vi "9205_UI.vi"(8 "error in (no error)":errorcluster, 11 "Node Ptr":T2 format="%.0x") -> (0 "error out":errorcluster)   [LabVIEW 2017, in "Modules.lvlib" / "9205.lvclass"]
uses:
  9205.lvclass
  <vilib>/NI Veristand/Custom Device API/Custom Device Item Ref.ctl
  RSI Module/SubPanel Command.ctl
  C:/Users/dbuck/Documents/GitHub/Scan-Engine-Custom-Device-Classes/Source/RSI Module/RSI Module.lvclass
  9205.lvclass/9205.ctl
  Range.ctl
  Terminal mode.ctl
  RSI Module/RSI Module.lvclass
  <vilib>/NI Veristand/Custom Device API/Custom Device API.lvlib
panel:
  in  "_Update Chan Settings":bool
  in  "_Update Ring Controls":bool
  in  "_Voltage Ranges":T1(array[ring])=[enum."+/- 10V", enum."+/- 10V", enum."+/- 10V", enum."+/- 10V", enum."+/- 10V", enum."+/- 10V", enum."+/- 10V", enum."+/- 10V", enum."+/- 10V", enum."+/- 10V", enum."+/- 10V", enum."+/- 10V", enum."+/- 10V", enum."+/- 10V", enum."+/- 10V", enum."+/- 10V", enum."+/- 10V", enum."+/- 10V", enum."+/- 10V", enum."+/- 10V", enum."+/- 10V", enum."+/- 10V", enum."+/- 10V", enum."+/- 10V", enum."+/- 10V", enum."+/- 10V", enum."+/- 10V", enum."+/- 10V", enum."+/- 10V", enum."+/- 10V", enum."+/- 10V", enum."+/- 10V"]
  in  "_Terminal Modes":enum8{"RSE", "NRSE", "DIFF"}[](array[ring])=[enum."RSE", enum."RSE", enum."RSE", enum."RSE", enum."RSE", enum."RSE", enum."RSE", enum."RSE", enum."RSE", enum."RSE", enum."RSE", enum."RSE", enum."RSE", enum."RSE", enum."RSE", enum."RSE", enum."RSE", enum."RSE", enum."RSE", enum."RSE", enum."RSE", enum."RSE", enum."RSE", enum."RSE", enum."RSE", enum."RSE", enum."RSE", enum."RSE", enum."RSE", enum."RSE", enum."RSE", enum."RSE"]
  out "_SupportedRanges":string[][](array[string])=[["+/- 10V", "+/- 5V", "+/- 1V", "+/- 200mV"], ["+/- 10V", "+/- 5V", "+/- 1V", "+/- 200mV"], ["+/- 10V", "+/- 5V", "+/- 1V", "+/- 200mV"], ["+/- 10V", "+/- 5V", "+/- 1V", "+/- 200mV"], ["+/- 10V", "+/- 5V", "+/- 1V", "+/- 200mV"], ["+/- 10V", "+/- 5V", "+/- 1V", "+/- 200mV"], ["+/- 10V", "+/- 5V", "+/- 1V", "+/- 200mV"], ["+/- 10V", "+/- 5V", "+/- 1V", "+/- 200mV"], ["+/- 10V", "+/- 5V", "+/- 1V", "+/- 200mV"], ["+/- 10V", "+/- 5V", "+/- 1V", "+/- 200mV"], ["+/- 10V", "+/- 5V", "+/- 1V", "+/- 200mV"], ["+/- 10V", "+/- 5V", "+/- 1V", "+/- 200mV"], ["+/- 10V", "+/- 5V", "+/- 1V", "+/- 200mV"], ["+/- 10V", "+/- 5V", "+/- 1V", "+/- 200mV"], ["+/- 10V", "+/- 5V", "+/- 1V", "+/- 200mV"], ["+/- 10V", "+/- 5V", "+/- 1V", "+/- 200mV"], ["+/- 10V", "+/- 5V", "+/- 1V", "+/- 200mV"], ["+/- 10V", "+/- 5V", "+/- 1V", "+/- 200mV"], ["+/- 10V", "+/- 5V", "+/- 1V", "+/- 200mV"], ["+/- 10V", "+/- 5V", "+/- 1V", "+/- 200mV"], ["+/- 10V", "+/- 5V", "+/- 1V", "+/- 200mV"], ["+/- 10V", "+/- 5V", "+/- 1V", "+/- 200mV"], ["+/- 10V", "+/- 5V", "+/- 1V", "+/- 200mV"], ["+/- 10V", "+/- 5V", "+/- 1V", "+/- 200mV"], ["+/- 10V", "+/- 5V", "+/- 1V", "+/- 200mV"], ["+/- 10V", "+/- 5V", "+/- 1V", "+/- 200mV"], ["+/- 10V", "+/- 5V", "+/- 1V", "+/- 200mV"], ["+/- 10V", "+/- 5V", "+/- 1V", "+/- 200mV"], ["+/- 10V", "+/- 5V", "+/- 1V", "+/- 200mV"], ["+/- 10V", "+/- 5V", "+/- 1V", "+/- 200mV"], ["+/- 10V", "+/- 5V", "+/- 1V", "+/- 200mV"], ["+/- 10V", "+/- 5V", "+/- 1V", "+/- 200mV"]]
  out "_SupportedTerminalModes":string[][](array[string])=[["RSE", "NRSE", "DIFF"], ["RSE", "NRSE", "DIFF"], ["RSE", "NRSE", "DIFF"], ["RSE", "NRSE", "DIFF"], ["RSE", "NRSE", "DIFF"], ["RSE", "NRSE", "DIFF"], ["RSE", "NRSE", "DIFF"], ["RSE", "NRSE", "DIFF"], ["RSE", "NRSE", ""], ["RSE", "NRSE", ""], ["RSE", "NRSE", ""], ["RSE", "NRSE", ""], ["RSE", "NRSE", ""], ["RSE", "NRSE", ""], ["RSE", "NRSE", ""], ["RSE", "NRSE", ""], ["RSE", "NRSE", "DIFF"], ["RSE", "NRSE", "DIFF"], ["RSE", "NRSE", "DIFF"], ["RSE", "NRSE", "DIFF"], ["RSE", "NRSE", "DIFF"], ["RSE", "NRSE", "DIFF"], ["RSE", "NRSE", "DIFF"], ["RSE", "NRSE", "DIFF"], ["RSE", "NRSE", ""], ["RSE", "NRSE", ""], ["RSE", "NRSE", ""], ["RSE", "NRSE", ""], ["RSE", "NRSE", ""], ["RSE", "NRSE", ""], ["RSE", "NRSE", ""], ["RSE", "NRSE", ""]]
  in  "Input Range":u16(ring) items=["+/- 10V", "+/- 5V", "+/- 1V", "+/- 200mV"]
  in  "Terminal Mode":u16(ring) items=["RSE", "NRSE", "DIFF"]
  in  "Channels":i32[](listbox)=[0]
  in  "Min Time Between Conversions":dbl[unit]=4e-06 caption="Minimum Time Between Conversions" min=4.5e-06 max=0.0015 step=2.5e-08
  in  "SubPanel Event":refnum<user-event>
  in  "Header":cluster{"Section Name":string}={"Section Name"="NI 9205 Settings"}
  # "Channel Configuration"
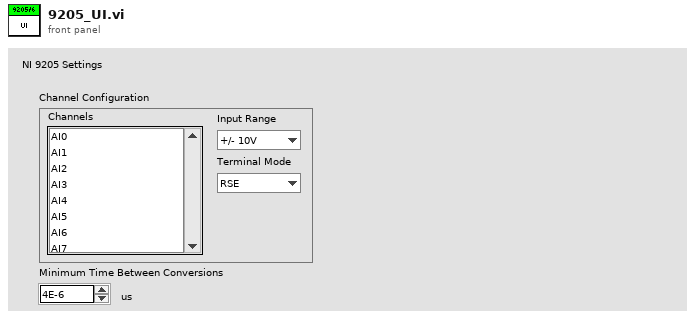
[diagram p1: front panel]
types:
  T1 = enum8{"+/- 10V", "+/- 5V", "+/- 1V", "+/- 200mV"}[]
  T2 = typedef "Custom Device API.lvlib/Custom Device Item Ref.ctl" = u64
  T3 = cluster{"NumChannels":u32, "FastestValidMinConvTime":dbl[unit]}
  T4 = typedef "Modules.lvlib/9205.lvclass/Channel Settings.ctl" = cluster{"Range":T5, "Terminal mode":T6}[]
  T5 = typedef "Modules.lvlib/9205.lvclass/Range.ctl" = u32
  T6 = typedef "Modules.lvlib/9205.lvclass/Terminal mode.ctl" = u32
  T7 = typedef "Modules.lvlib/RSI Module.lvclass/Module Models.ctl" = enum16{"Empty", "NI 9201", "NI 9203", "NI 9205", "NI 9206", "NI 9207", "NI 9208", "NI 9211", "NI 9212", "NI 9213", "NI 9214", "NI 9215", "NI 9217", "NI 9219", "NI 9220", "NI 9221", "NI 9222", "NI 9223", "NI 9225", "NI 9227", "NI 9229", "NI 9233", "NI 9234", "NI 9235", "NI 9236", "NI 9237", "NI 9239", "NI 9242", "NI 9244", "NI 9263", "NI 9264", "NI 9265", "NI 9269", "NI 9375", "NI 9401", "NI 9402", "NI 9403", "NI 9411", "NI 9421", "NI 9422", "NI 9423", "NI 9425", "NI 9426", "NI 9435", "NI 9437", "NI 9472", "NI 9474", "NI 9475", "NI 9476", "NI 9477", "NI 9478", "NI 9481", "NI 9482", "NI 9485"}
  T8 = typedef "Modules.lvlib/RSI Module.lvclass/SubPanel Command.ctl" = enum16{"Stop"}
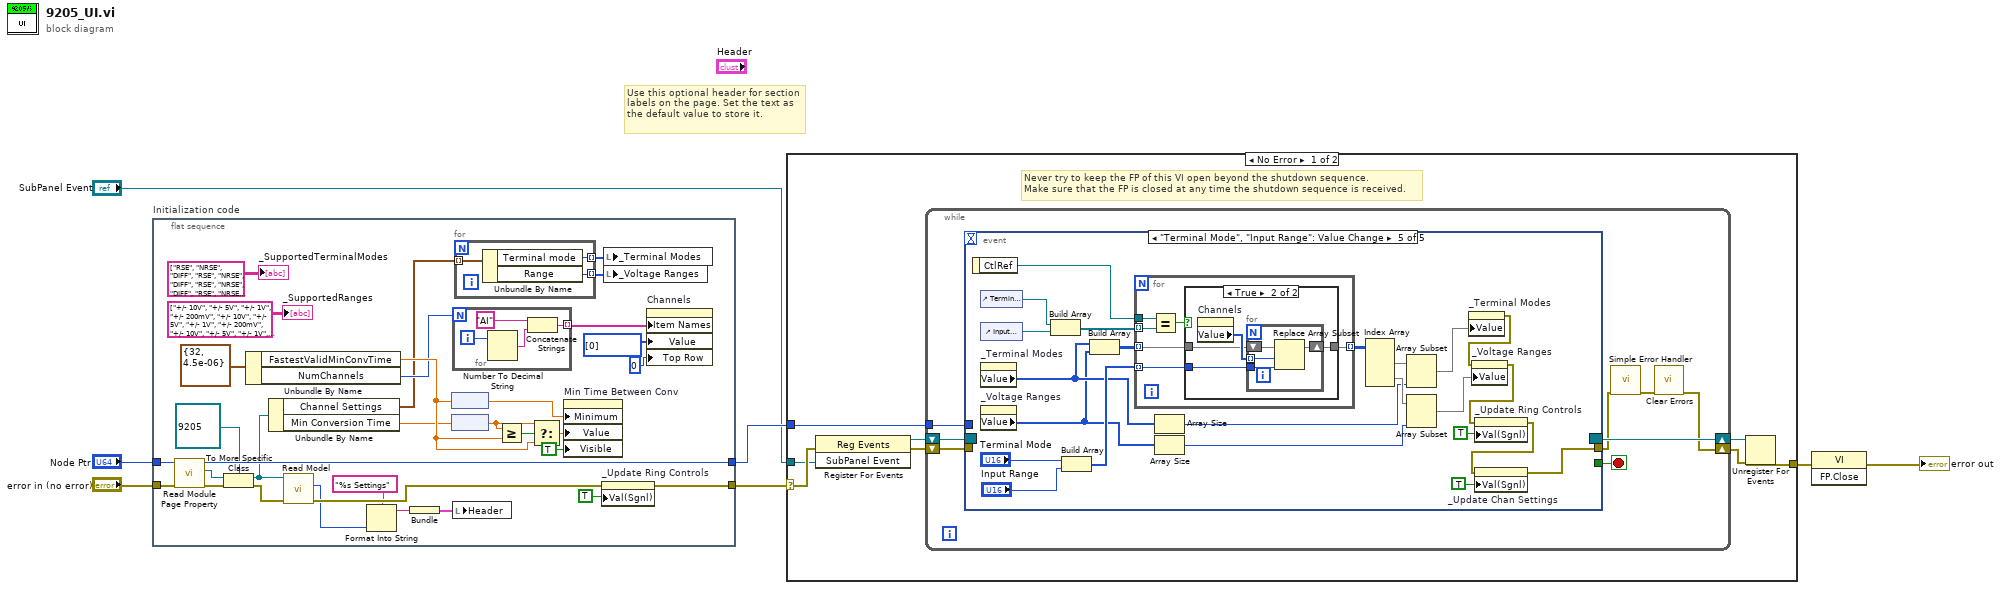
[diagram p0: block diagram]
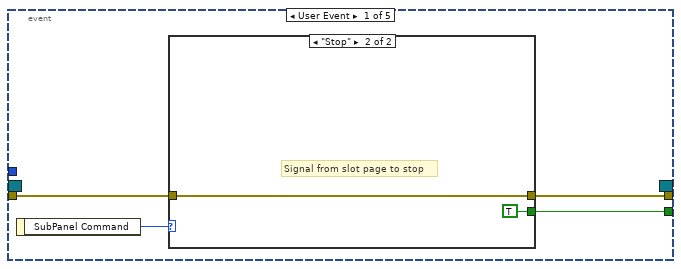
[diagram p2: hidden frame]
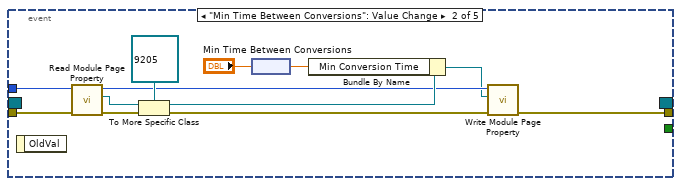
[diagram p4: hidden frame]
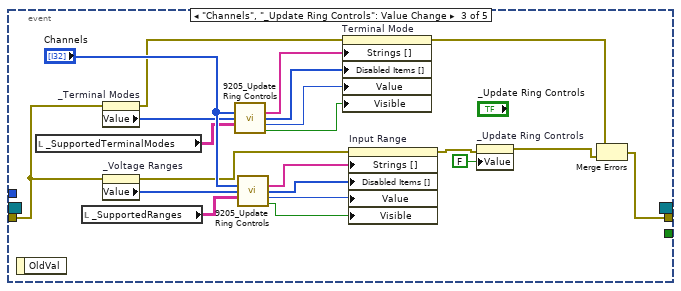
[diagram p5: hidden frame]
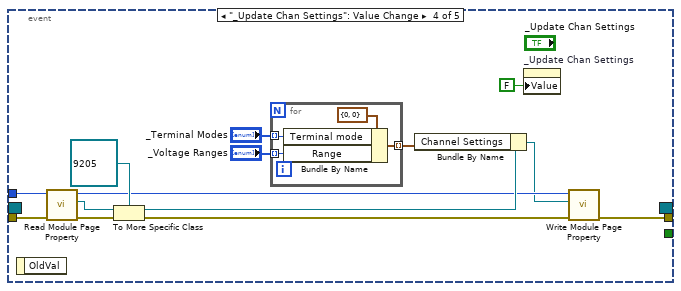
[diagram p6: hidden frame]
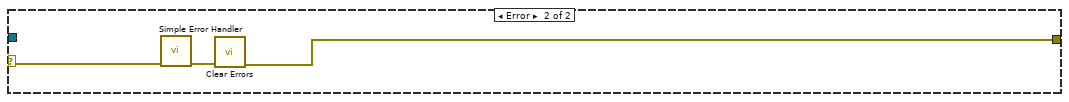
[diagram p8: hidden frame]
diagram:
  # "Use this optional header for section labels on the page. Set the text as the default value to store it."
  n1 = flat-sequence "Initialization code" {
    tunnel: "error in (no error)" -> [w38]
    tunnel: "Node Ptr" -> [w39]
    tunnel: [w15] -> w1
    tunnel: [w37] -> w4
    frame #0 {
      n2 = call "Read Module Page Property.vi"("error in (no error)"=w38, "Node Ptr In"=w39) -> ("error out"=w36:errorcluster, "RSI Module"=w34:refnum<class "RSI Module.lvclass">, "Node Ptr Out"=w37:T2)  [unwired: 7 in]
      n3 = To More Specific Class(target class=refnum<class "9205.lvclass"> refnum ("9205 in"), reference=w34, error in=w36) -> (specific class reference=w14:refnum<class "9205.lvclass">, error out=w13:errorcluster)
      n4 = Unbundle By Name(T3 {"NumChannels"=32, "FastestValidMinConvTime"=4.5e-06} ("cRIO-920x ModuleSpecificSettings")) -> ("FastestValidMinConvTime"=w27:dbl[unit], "NumChannels"=w26:u32)
      n5 = Unbundle By Name(w14) -> ("Channel Settings"=w16:T4, "Min Conversion Time"=w24:dbl)
      n6 = call "Read Model.vi"("error in (no error)"=w13, "RSI Module in"=w14) -> ("error out"=w12:errorcluster, "Model"=w10:T7)  [unwired: 7 in, 1 out]
      n7 = Format Into String(format string="%s Settings", w10) -> (resulting string=w8:string)  [unwired: 2 in, 1 out]
      n8 = Bundle(w8) -> (w11:cluster{string})  [unwired: 1 in]
      n9 = node(w27) -> (w29:dbl)
      n10 = node(w24) -> (w23:dbl[unit])
      n11 = for {
        N: w26 -> [_]
        tunnel: [w43] -> w32 mode=indexing
        i -> [w45]
        n12 = Number To Decimal String(number=w45) -> (decimal integer string=w44:string)  [unwired: 1 out]
        n13 = Concatenate Strings("AI", w44) -> (w43:string)
      }
      n14 = local write "Header"(w11) -> ()
      n15 = for {
        tunnel: w16 -> [w42] mode=indexing
        tunnel: [w41] -> w22 mode=indexing
        tunnel: [w40] -> w21 mode=indexing
        n16 = Unbundle By Name(w42) -> ("Terminal mode"=w41:T6, "Range"=w40:T5)
      }
      n17 = Greater Or Equal?(x=w23, y=w27) -> (x >= y?=w31:bool)
      n18 = Select(t=w23, s=w31, f=w27) -> (s? t:f=w30:dbl[unit])
      n19 = property on="Min Time Between Conv" class="DigNum (strict)"("Minimum"=w29, "Value"=w30, "Visible"=TRUE) -> ()  [unwired: 2 in, 2 out]
      n20 = property on="_Update Ring Controls" class="Bool (strict)"(error in=w12, "Val(Sgnl)"=TRUE ("Value (Signaling)")) -> (error out=w15:errorcluster)  [unwired: 1 in, 1 out]
      n21 = local write "_Terminal Modes"(w22) -> ()
      n22 = local write "_Voltage Ranges"(w21) -> ()
      n23 = property on="Channels" class="LstBox (strict)"("Item Names"=w32, "Value"=i32[] [0] ("Channels"), "Top Row"=0) -> ()  [unwired: 2 in, 2 out]
      "_SupportedTerminalModes" <- string[][] [["RSE", "NRSE", "DIFF"], ["RSE", "NRSE", "DIFF"], ["RSE", "NRSE", "DIFF"], ["RSE", "NRSE", "DIFF"], ["RSE", "NRSE", "DIFF"], ["RSE", "NRSE", "DIFF"], ["RSE", "NRSE", "DIFF"], ["RSE", "NRSE", "DIFF"], ["RSE", "NRSE", ""], ["RSE", "NRSE", ""], ["RSE", "NRSE", ""], ["RSE", "NRSE", ""], ["RSE", "NRSE", ""], ["RSE", "NRSE", ""], ["RSE", "NRSE", ""], ["RSE", "NRSE", ""], ["RSE", "NRSE", "DIFF"], ["RSE", "NRSE", "DIFF"], ["RSE", "NRSE", "DIFF"], ["RSE", "NRSE", "DIFF"], ["RSE", "NRSE", "DIFF"], ["RSE", "NRSE", "DIFF"], ["RSE", "NRSE", "DIFF"], ["RSE", "NRSE", "DIFF"], ["RSE", "NRSE", ""], ["RSE", "NRSE", ""], ["RSE", "NRSE", ""], ["RSE", "NRSE", ""], ["RSE", "NRSE", ""], ["RSE", "NRSE", ""], ["RSE", "NRSE", ""], ["RSE", "NRSE", ""]] ("Terminal Modes")
      "_SupportedRanges" <- string[][] [["+/- 10V", "+/- 5V", "+/- 1V", "+/- 200mV"], ["+/- 10V", "+/- 5V", "+/- 1V", "+/- 200mV"], ["+/- 10V", "+/- 5V", "+/- 1V", "+/- 200mV"], ["+/- 10V", "+/- 5V", "+/- 1V", "+/- 200mV"], ["+/- 10V", "+/- 5V", "+/- 1V", "+/- 200mV"], ["+/- 10V", "+/- 5V", "+/- 1V", "+/- 200mV"], ["+/- 10V", "+/- 5V", "+/- 1V", "+/- 200mV"], ["+/- 10V", "+/- 5V", "+/- 1V", "+/- 200mV"], ["+/- 10V", "+/- 5V", "+/- 1V", "+/- 200mV"], ["+/- 10V", "+/- 5V", "+/- 1V", "+/- 200mV"], ["+/- 10V", "+/- 5V", "+/- 1V", "+/- 200mV"], ["+/- 10V", "+/- 5V", "+/- 1V", "+/- 200mV"], ["+/- 10V", "+/- 5V", "+/- 1V", "+/- 200mV"], ["+/- 10V", "+/- 5V", "+/- 1V", "+/- 200mV"], ["+/- 10V", "+/- 5V", "+/- 1V", "+/- 200mV"], ["+/- 10V", "+/- 5V", "+/- 1V", "+/- 200mV"], ["+/- 10V", "+/- 5V", "+/- 1V", "+/- 200mV"], ["+/- 10V", "+/- 5V", "+/- 1V", "+/- 200mV"], ["+/- 10V", "+/- 5V", "+/- 1V", "+/- 200mV"], ["+/- 10V", "+/- 5V", "+/- 1V", "+/- 200mV"], ["+/- 10V", "+/- 5V", "+/- 1V", "+/- 200mV"], ["+/- 10V", "+/- 5V", "+/- 1V", "+/- 200mV"], ["+/- 10V", "+/- 5V", "+/- 1V", "+/- 200mV"], ["+/- 10V", "+/- 5V", "+/- 1V", "+/- 200mV"], ["+/- 10V", "+/- 5V", "+/- 1V", "+/- 200mV"], ["+/- 10V", "+/- 5V", "+/- 1V", "+/- 200mV"], ["+/- 10V", "+/- 5V", "+/- 1V", "+/- 200mV"], ["+/- 10V", "+/- 5V", "+/- 1V", "+/- 200mV"], ["+/- 10V", "+/- 5V", "+/- 1V", "+/- 200mV"], ["+/- 10V", "+/- 5V", "+/- 1V", "+/- 200mV"], ["+/- 10V", "+/- 5V", "+/- 1V", "+/- 200mV"], ["+/- 10V", "+/- 5V", "+/- 1V", "+/- 200mV"]] ("Ranges")
    }
  }
  n24 = case shown="No Error" w1 {
    selector: w1 -> [w48 w161]
    tunnel: [w52 w159] -> w7
    tunnel: w4 -> [w49 _]
    tunnel: "SubPanel Event" -> [w47 _]
    frame No Error {
      # "Never try to keep the FP of this VI open beyond the shutdown sequence.\nMake sure that the FP is closed at any time the shutdown sequence is received."
      n25 = register-events(error in=w48, w47) -> (reference out=w50:refnum<event-registration>, error out=w51:errorcluster)  [unwired: 1 in]
      n26 = while {
        tunnel: w49 -> [w58]
        shift-right: [w55] -> w53
        shift-left: w51 -> [w61]
        shift-right: [w62] -> w54
        shift-left: w50 -> [w60]
        stop <- w59 stop-if-true
        n27 = event shown="[4] \"Terminal Mode\", \"Input Range\": Value Change" {
          selector: w60 -> [_ _ _ _ _]
          dyn-events: [_ _ _ _ _] -> w62
          timeout: _ -> [_ _ _ _ _]
          tunnel: w61 -> [w65 w73 w88 w108 _]
          tunnel: [w64 _ _ _ _] -> w59
          tunnel: [w63 w72 w82 w107 w121] -> w57
          tunnel: w58 -> [_ w74 _ w109 _]
          event User Event {
            n28 = event-data() -> ("SubPanel Command"=w66:T8)  [unwired: 1 out]
            n29 = case shown="\"Stop\"" w66 {
              tunnel: w65 -> [w67 w68]
              tunnel: [w67 w68] -> w63
              tunnel: [_ TRUE] -> w64
              frame Default {
              }
              frame "Stop" {
                # "Signal from slot page to stop"
              }
            }
          }
          event "Min Time Between Conversions": Value Change {
            n30 = event-data() -> ()  [unwired: 2 out]
            n31 = call "Read Module Page Property.vi"("error in (no error)"=w73, "Node Ptr In"=w74) -> ("error out"=w79:errorcluster, "RSI Module"=w80:refnum<class "RSI Module.lvclass">, "Node Ptr Out"=w76:T2)  [unwired: 7 in]
            n32 = To More Specific Class(target class=refnum<class "9205.lvclass"> refnum ("9205 in"), reference=w80, error in=w79) -> (specific class reference=w78:refnum<class "9205.lvclass">, error out=w77:errorcluster)
            n33 = node("Min Time Between Conversions") -> (w70:dbl)
            n34 = Bundle By Name(cluster=w78, "Min Conversion Time"=w70) -> (w75:refnum<class "9205.lvclass">)
            n35 = call "Write Module Page Property.vi"("error in (no error)"=w77, "RSI Module"=w75, "Node Ptr In"=w76) -> ("error out"=w72:errorcluster)  [unwired: 6 in, 2 out]
          }
          event "Channels", "_Update Ring Controls": Value Change {
            n36 = event-data() -> ()  [unwired: 2 out]
            n37 = local read "_SupportedTerminalModes"() -> (w99:string[][])
            n38 = local read "_SupportedRanges"() -> (w98:string[][])
            n39 = property on="_Terminal Modes" class="Arr (strict)"(error in=w88) -> (error out=w86:errorcluster, "Value"=w101:enum8{"RSE", "NRSE", "DIFF"}[])  [unwired: 1 in, 1 out]
            n40 = property on="_Voltage Ranges" class="Arr (strict)"(error in=w88) -> (error out=w87:errorcluster, "Value"=w100:T1)  [unwired: 1 in, 1 out]
            n41 = call "9205_Update Ring Controls.vi"("SelectedChannels"="Channels", "ChannelConfig"=w101, "SupportedModes"=w99) -> ("Strings out"=w97:string[], "Disabled Items out"=w95:i32[], "Value out"=w94:u8, "Visible out"=w93:bool)  [unwired: 9 in]
            n42 = call "9205_Update Ring Controls.vi"("SelectedChannels"="Channels", "ChannelConfig"=w100, "SupportedModes"=w98) -> ("Strings out"=w96:string[], "Disabled Items out"=w92:i32[], "Value out"=w91:u8, "Visible out"=w90:bool)  [unwired: 9 in]
            n43 = property on="Terminal Mode" class="Ring (strict)"(error in=w86, "Strings []"=w97, "Disabled Items []"=w95, "Value"=w94, "Visible"=w93) -> (error out=w83:errorcluster)  [unwired: 1 in, 1 out]
            n44 = property on="Input Range" class="Ring (strict)"(error in=w87, "Strings []"=w96, "Disabled Items []"=w92, "Value"=w91, "Visible"=w90) -> (error out=w85:errorcluster)  [unwired: 1 in, 1 out]
            n45 = property on="_Update Ring Controls" class="Bool (strict)"(error in=w85, "Value"=FALSE ("_Update Ring Controls 2")) -> (error out=w84:errorcluster)  [unwired: 1 in, 1 out]
            n46 = Merge Errors(w83, w84) -> (w82:errorcluster)
          }
          event "_Update Chan Settings": Value Change {
            n47 = event-data() -> ()  [unwired: 2 out]
            n48 = call "Read Module Page Property.vi"("error in (no error)"=w108, "Node Ptr In"=w109) -> ("error out"=w114:errorcluster, "RSI Module"=w115:refnum<class "RSI Module.lvclass">, "Node Ptr Out"=w111:T2)  [unwired: 7 in]
            n49 = To More Specific Class(target class=refnum<class "9205.lvclass"> refnum ("9205 in"), reference=w115, error in=w114) -> (specific class reference=w113:refnum<class "9205.lvclass">, error out=w112:errorcluster)
            n50 = for {
              tunnel: "_Terminal Modes" -> [w118] mode=indexing
              tunnel: "_Voltage Ranges" -> [w119] mode=indexing
              tunnel: [w117] -> w103 mode=indexing
              n51 = Bundle By Name(cluster=cluster{"Range":T5, "Terminal mode":T6} {"Range"=0, "Terminal mode"=0} ("element"), "Terminal mode"=w118, "Range"=w119) -> (w117:cluster{"Range":T5, "Terminal mode":T6})
            }
            n52 = Bundle By Name(cluster=w113, "Channel Settings"=w103) -> (w110:refnum<class "9205.lvclass">)
            n53 = property on="_Update Chan Settings" class="Bool (strict)"("Value"=FALSE ("_Update Values")) -> ()  [unwired: 2 in, 2 out]
            n54 = call "Write Module Page Property.vi"("error in (no error)"=w112, "RSI Module"=w110, "Node Ptr In"=w111) -> ("error out"=w107:errorcluster)  [unwired: 6 in, 2 out]
          }
          event "Terminal Mode", "Input Range": Value Change {
            n55 = event-data() -> ("CtlRef"=w137:refnum<vi>)  [unwired: 1 out]
            n56 = control-ref of="Terminal Mode"() -> (w140:refnum<vi>)
            n57 = control-ref of="Input Range"() -> (w139:refnum<vi>)
            n58 = property on="_Terminal Modes" class="Arr (strict)"() -> ("Value"=w135:enum8{"RSE", "NRSE", "DIFF"}[])  [unwired: 2 in, 2 out]
            n59 = property on="_Voltage Ranges" class="Arr (strict)"() -> ("Value"=w134:T1)  [unwired: 2 in, 2 out]
            n60 = Build Array(w140, w139) -> (w138:refnum<vi>[])
            n61 = Build Array("Terminal Mode", "Input Range") -> (w143:u16[])
            n62 = Build Array(w135, w134) -> (w136:u8[][])
            n63 = for {
              tunnel: w143 -> [w149] mode=indexing
              tunnel: w136 -> [w148] mode=indexing
              tunnel: [w147] -> w131 mode=indexing
              tunnel: w138 -> [w145] mode=indexing
              tunnel: w137 -> [w144]
              n64 = Equal?(x=w144, y=w145) -> (x = y?=w146:bool)
              n65 = case shown="True" w146 {
                tunnel: w149 -> [_ w153]
                tunnel: w148 -> [w150 w152]
                tunnel: [w150 w151] -> w147
                frame False {
                }
                frame True {
                  n66 = property on="Channels" class="LstBox (strict)"() -> ("Value"=w154:i32[])  [unwired: 2 in, 2 out]
                  n67 = for {
                    tunnel: w153 -> [w157]
                    tunnel: w154 -> [w155] mode=indexing
                    shift-right: [w156] -> w151
                    shift-left: w152 -> [w158]
                    n68 = Replace Array Subset(array=w158, new element=w157, index=w155) -> (w156:u8[])
                  }
                }
              }
            }
            n69 = Array Size(array=w135) -> (size(s)=w130:i32)
            n70 = Array Size(array=w134) -> (size(s)=w129:i32)
            n71 = Index Array(array=w131) -> (element #1=w132:u8[], element #2=w133:u8[])  [unwired: 4 in]
            n72 = Array Subset(array=w132, length=w130) -> (w127:u8[])  [unwired: 1 in]
            n73 = Array Subset(array=w133, length=w129) -> (w126:u8[])  [unwired: 1 in]
            n74 = property on="_Terminal Modes" class="Arr (strict)"("Value"=w127) -> (error out=w128:errorcluster)  [unwired: 2 in, 1 out]
            n75 = property on="_Voltage Ranges" class="Arr (strict)"(error in=w128, "Value"=w126) -> (error out=w124:errorcluster)  [unwired: 1 in, 1 out]
            n76 = property on="_Update Ring Controls" class="Bool (strict)"(error in=w124, "Val(Sgnl)"=TRUE ("Value (Signaling)")) -> (error out=w122:errorcluster)  [unwired: 1 in, 1 out]
            n77 = property on="_Update Chan Settings" class="Bool (strict)"(error in=w122, "Val(Sgnl)"=TRUE ("Value (Signaling)")) -> (error out=w121:errorcluster)  [unwired: 1 in, 1 out]
          }
        }
        n78 = call <vilib>:"Simple Error Handler.vi"("error in (no error)"=w57) -> ("error out"=w56:errorcluster)  [unwired: 1 in, 7 out]
        n79 = call <vilib>:"Clear Errors.vi"("error in (no error)"=w56) -> ("error out"=w55:errorcluster)  [unwired: 1 in, 5 out]
      }
      n80 = Unregister For Events(event registration refnum=w54, error in=w53) -> (error out=w52:errorcluster)
    }
    frame Error {
      n81 = call <vilib>:"Simple Error Handler.vi"("error in (no error)"=w161) -> ("error out"=w160:errorcluster)  [unwired: 1 in, 7 out]
      n82 = call <vilib>:"Clear Errors.vi"("error in (no error)"=w160) -> ("error out"=w159:errorcluster)  [unwired: 1 in, 5 out]
    }
  }
  n83 = invoke class="VI" method="FP.Close"(error in=w7) -> (error out=→"error out":errorcluster)  [unwired: 2 in, 2 out]
